vi "Write loopInternalConfig.vi"(8 "error in (no error)":errorcluster, 10 "LoopInternalConfig.lvclass":refnum<class "LoopInternalConfig.lvclass">, 11 "LoopTimer in":refnum<class "LoopTimer.lvclass">) -> (0 "error out":errorcluster, 3 "LoopTimer out":refnum<class "LoopTimer.lvclass">)   [LabVIEW 2013, in "ComponentData.lvlib" / "LoopTimer.lvclass"]
uses:
  <userlib>/Common/Component/common_application/RT/ComponentData/LoopTimer/LoopTimer.lvclass
  <userlib>/Common/Component/common_application/RT/ComponentData/ConfigurationHandler/LoopInternalConfig/LoopInternalConfig.lvclass
  <userlib>/Common/Component/common_application/RT/ComponentData/LoopTimer/LoopTimer.lvclass/LoopTimer.ctl
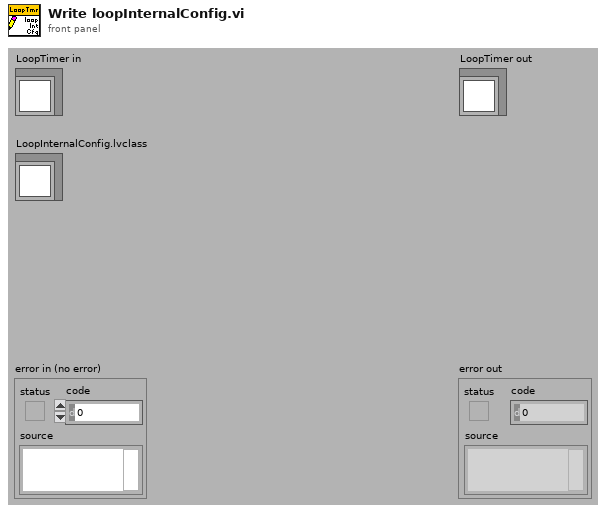
[diagram p1: front panel]
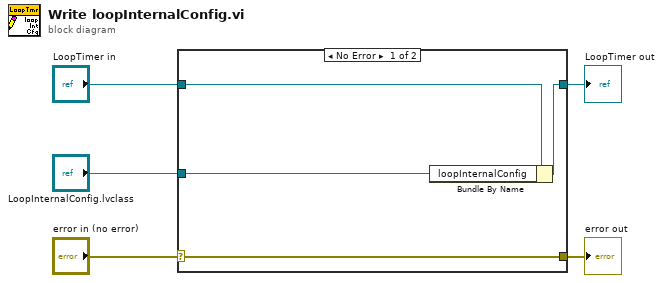
[diagram p0: block diagram]
diagram:
  n1 = case shown="No Error" "error in (no error)" {
    selector: "error in (no error)" -> [w9 w10]
    tunnel: [w9 w10] -> w4
    tunnel: [w7 w11] -> w2
    tunnel: "LoopTimer in" -> [w8 w11]
    tunnel: "LoopInternalConfig.lvclass" -> [w6 _]
    frame No Error {
      n2 = Bundle By Name(cluster=w8, "loopInternalConfig"=w6) -> (w7:refnum<class "LoopTimer.lvclass">)
    }
    frame Error {
    }
  }
  "error out" <- w4
  "LoopTimer out" <- w2
